vi "HC-SR04.vi"(8 "Error In":errorcluster, 9 "Echo Pin (DI)":u8, 10 "Trig":u8, 11 "LINX Resource":T1) -> (0 "Error Out":errorcluster, 1 "Inches":dbl, 2 "Centimeters":dbl, 3 "LINX Resource":T1)   [LabVIEW 2019, in "LMH-LINX.lvlib" / "Ultrasonic.lvlib"]
doc: "Read distance using the HC-SR04 ultrasonic distance sensor."
uses:
  <vilib>/MakerHub/LINX/Public/Sensors/Distance/Ultrasonic/Ultrasonic.lvlib
  <vilib>/MakerHub/LINX/Private/Type Defs/LINX Ref.ctl
  <vilib>/MakerHub/LINX/Private/Type Defs/Platform.ctl
  <vilib>/MakerHub/LINX/Private/Type Defs/Interface.ctl
  <vilib>/MakerHub/LINX/Private/Device/Type Defs/LINX Device Config.ctl
  <vilib>/MakerHub/LINX/Private/Device/Type Defs/TCP Config.ctl
  <vilib>/MakerHub/LINX/Private/Device/Type Defs/Channels.ctl
  <vilib>/MakerHub/LINX/LMH-LINX.lvlib
  <vilib>/MakerHub/LINX/Private/Device/Device.lvlib
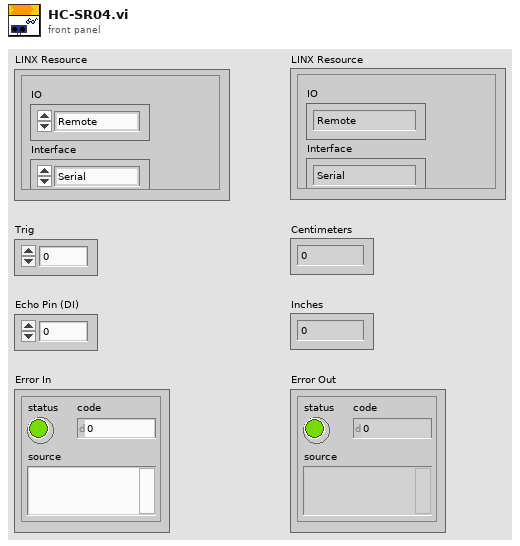
[diagram p1: front panel]
types:
  T1 = typedef "LMH-LINX.lvlib/LINX Ref.ctl" = cluster{"IO":T2, "Interface":T3, "LINX Device Config":T4}
  T2 = typedef "LMH-LINX.lvlib/Platform.ctl" = enum16{"Remote", "Local"}
  T3 = typedef "LMH-LINX.lvlib/Interface.ctl" = enum16{"Serial", "TCP"}
  T4 = typedef "LMH-LINX.lvlib/Device.lvlib/LINX Device Config.ctl" = cluster{"Interface":T3, "COM Port":refnum<visa-resource-name>, "TCP Configuration":T5, "Device Family":u8, "Device ID":u8, "Device Name":string, "TCP Ref":refnum<k5>, "Channels":T6}
  T5 = typedef "LMH-LINX.lvlib/Device.lvlib/TCP Config.ctl" = cluster{"IP Address":string, "Port":u16}
  T6 = typedef "LMH-LINX.lvlib/Channels.ctl" = cluster{"DI":u8[], "DO":u8[], "AI":u8[], "AO":u8[], "PWM":u8[], "QE":u8[], "UART":u8[], "I2C 2":u8[], "SPI":u8[], "CAN":u8[], "Servo":u8[], "AI Ref (V)":dbl, "AI Resolution (Bits)":u8, "AO Ref (V)":dbl, "AO Resolution (Bits)":u8}
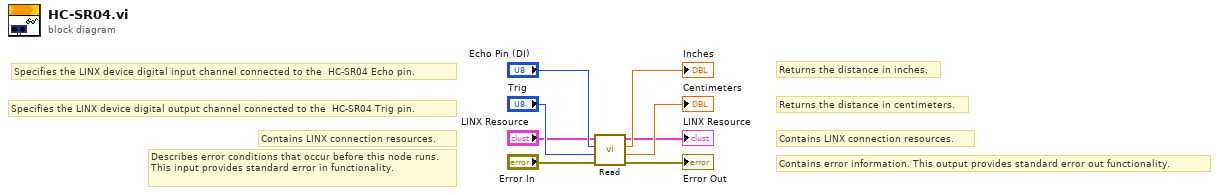
[diagram p0: block diagram]
diagram:
  # "Specifies the LINX device digital output channel connected to the  HC-SR04 Trig pin."
  # "Returns the distance in centimeters."
  # "Returns the distance in inches."
  # "Specifies the LINX device digital input channel connected to the  HC-SR04 Echo pin."
  # "Contains LINX connection resources."
  # "Contains error information. This output provides standard error out functionality."
  # "Contains LINX connection resources."
  # "Describes error conditions that occur before this node runs. This input provides standard error in functionality."
  n1 = call <vilib>:"Read.vi"("Error In"="Error In", "DO Channel"="Trig", "DI Channel"="Echo Pin (DI)", "LINX Resource"="LINX Resource") -> ("Error Out"=→"Error Out":errorcluster, "Centimeters"=→"Centimeters":dbl, "Inches"=→"Inches":dbl, "LINX Resource"=→"LINX Resource":T1)  [unwired: 4 in]
